vi "TimerCalcMilis.vi"(6 "Active":bool, 9 "ElapsedTime in":u32, 10 "Timeout [ms]":u32, 11 "timeOfLastCall":u32) -> (1 "ElapsedTime out":u32, 2 "Done":bool, 3 "now":u32)   [LabVIEW 2024]
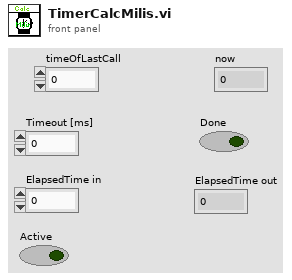
[diagram p1: front panel]
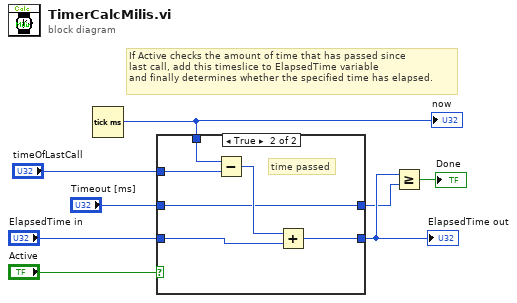
[diagram p0: block diagram]
diagram:
  # "If Active checks the amount of time that has passed since\nlast call, add this timeslice to ElapsedTime variable \nand finally determines whether the specified time has elapsed."
  n1 = Tick Count (ms)() -> (millisecond timer value=w1:u32)
  "now" <- w1
  n2 = case shown="True" "Active" {
    tunnel: w1 -> [_ w16]
    tunnel: "ElapsedTime in" -> [w10 w15]
    tunnel: "Timeout [ms]" -> [w9 w11]
    tunnel: "timeOfLastCall" -> [_ w13]
    tunnel: [w10 w12] -> w4
    tunnel: [w9 w11] -> w3
    frame False {
    }
    frame True {
      # "time passed"
      n3 = Subtract(x=w16, y=w13) -> (x-y=w14:u32)
      n4 = Add(x=w14, y=w15) -> (x+y=w12:u32)
    }
  }
  "ElapsedTime out" <- w4
  n5 = Greater Or Equal?(x=w4, y=w3) -> (x >= y?=→"Done":bool)
